vi "RUSHDriveTrain.vi"(0 "Servo Positions":T1={"Shifting"={"Right Servo High"=145.0, "Right Servo Low"=110.0, "Left Servo High"=70.0, "Left Servo Low"=110.0}, "Breaking"={"Coast Position"=0.0, "Break Position"=0.0}}, 5 "Low Gear + Brake":bool, 7 "Low Gear":bool, 9 "LeftJoystick":dbl, 11 "RightJoystick":dbl) -> (4 "Braking Servo":dbl, 6 "Left Drive":dbl, 8 "Right Drive":dbl, 10 "Left Servo":dbl, 15 "Right Servo":dbl)   [LabVIEW 2012]
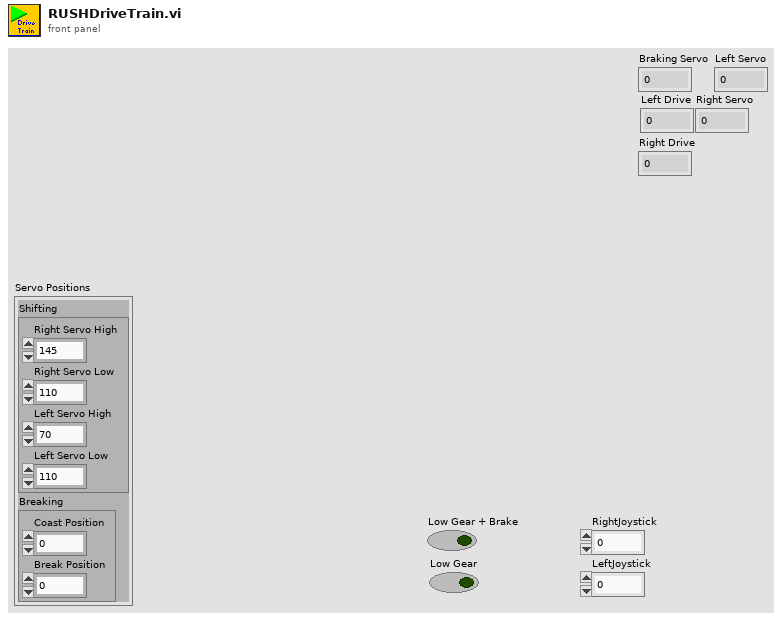
[diagram p1: front panel]
types:
  T1 = cluster{"Shifting":cluster{"Right Servo High":dbl, "Right Servo Low":dbl, "Left Servo High":dbl, "Left Servo Low":dbl}, "Breaking":cluster{"Coast Position":dbl, "Break Position":dbl}}
  T2 = cluster{"Right Servo High":dbl, "Right Servo Low":dbl, "Left Servo High":dbl, "Left Servo Low":dbl}
  T3 = cluster{"Coast Position":dbl, "Break Position":dbl}
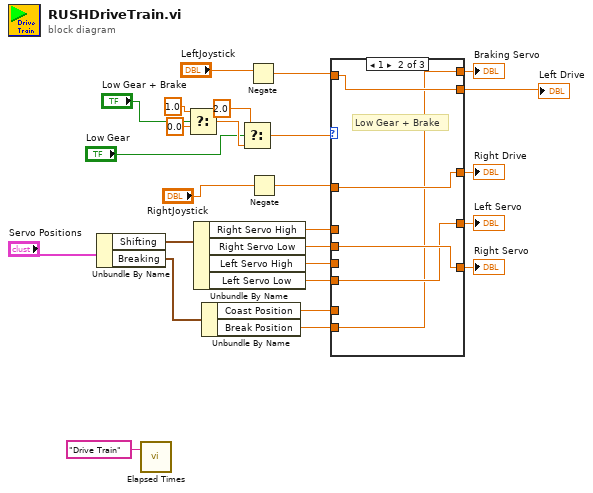
[diagram p0: block diagram]
diagram:
  n1 = Unbundle By Name("Servo Positions") -> ("Shifting"=w15:T2, "Breaking"=w13:T3)
  n2 = call "Elapsed Times.vi"("Call Name"="Drive Train") -> ()  [unwired: 2 in, 1 out]
  n3 = Select(t=1.0, s="Low Gear + Brake", f=0.0 ("t")) -> (s? t:f=w24:dbl)
  n4 = Unbundle By Name(w15) -> ("Right Servo High"=w7:dbl, "Right Servo Low"=w8:dbl, "Left Servo High"=w9:dbl, "Left Servo Low"=w10:dbl)
  n5 = Unbundle By Name(w13) -> ("Coast Position"=w11:dbl, "Break Position"=w12:dbl)
  n6 = Select(t=2.0, s="Low Gear", f=w24) -> (s? t:f=w22:dbl)
  n7 = Negate(x="LeftJoystick") -> (-x=w21:dbl)
  n8 = Negate(x="RightJoystick") -> (-x=w20:dbl)
  n9 = case shown="1" w22 {
    tunnel: w20 -> [w31 w36 w41]
    tunnel: [w31 w36 w41] -> w4
    tunnel: [w30 w35 w40] -> w5
    tunnel: [w28 w33 w38] -> w3
    tunnel: [w27 w34 w39] -> w2
    tunnel: w21 -> [w30 w35 w40]
    tunnel: [w29 w32 w37] -> w6
    tunnel: w12 -> [_ w32 _]
    tunnel: w11 -> [w29 _ w37]
    tunnel: w10 -> [_ w33 w38]
    tunnel: w9 -> [w28 _ _]
    tunnel: w8 -> [_ w34 w39]
    tunnel: w7 -> [w27 _ _]
    frame 0, Default {
      # "High Gear"
    }
    frame 1 {
      # "Low Gear + Brake"
    }
    frame 2 {
      # "Low Gear"
    }
  }
  "Braking Servo" <- w6
  "Left Drive" <- w5
  "Right Drive" <- w4
  "Left Servo" <- w3
  "Right Servo" <- w2
